vi "VI Linearisierung v2.vi"() -> ()   [LabVIEW 2020, in "Linearisierung v2.lvlib"] (continued)
                      n1878 = call "Komponentenindex aus SPAN.vi"("Component Index in"=w3418, "SPAN Idx in (Eingang)"=w3419, "SpanInletClusterArray in (Eingang)"=w3420) -> ("Component Index out"=w3403:i32, "SPAN Idx out"=w3404:i32, "Komponenten Index"=w3417:u16)  [unwired: 5 in, 1 out]
                      n1879 = Bundle("SPAN Idx out"=w3404, "Component Index out"=w3403) -> (w3402:T219)  [unwired: 1 in]
                      n1880 = Equal?(x=w3413, y=w3412) -> (x = y?=w3406:bool)
                      n1881 = Bundle(w3413, w3402) -> (w3405:T220)  [unwired: 1 in]
                      n1882 = Bundle(w3406, w3406, "Gesamtkonzentration"=w3408, "höchste Konzentration Teilkomponente"=w3407) -> (w3409:T221)  [unwired: 1 in]
                      n1883 = call "Stufen abfragen Tabelle setzen und auslesen.vi"("E/A Cluster"=w3409, "Ausgabetabelle (Eingang)"=w3410, "GD Cluster"=w3414, "Eingabetabelle (Eingang)"=w3411, "Fehler (Eingang, kein Fehler)"=w3421, "Komponente in"=w3417, "Index Cluster"=w3405, "GD in"=w3416) -> ("Fehler (Ausgang)"=w3415:errorcluster, "EGAK out"=w3422:T26[], "Stufen Tabellen out"=w3423:string[][])  [unwired: 1 out]
                    }
                  }
                }
                n1884 = Decrement(x=w3324) -> ()  [unwired: 1 out]
                n1885 = call "Komponentenindex aus SPAN.vi"("Component Index in"=w3301, "SPAN Idx in (Eingang)"=w3321, "SpanInletClusterArray in (Eingang)"=w3322) -> ("Summenformel"=w3305:T12)  [unwired: 5 in, 3 out]
                n1886 = call "set Tables Flag from SPANIdx.vi"("SPAN Idx"=w3302) -> ("set Tables"=w3304:bool)  [unwired: 10 in]
                n1887 = property class="Tbl (strikt)"(reference=w3357, "Value"=w3360) -> (error out=w3362:errorcluster)  [unwired: 1 in, 1 out]
                n1888 = property class="Arr (strikt)"(reference=w3367, error in=w3334, "Value"=w3359) -> (error out=w3361:errorcluster)  [unwired: 1 out]
                n1889 = property class="Str (strikt)"(reference=w3325, "Value"=w3305) -> (error out=w3315:errorcluster)  [unwired: 1 in, 1 out]
                n1890 = flat-sequence {
                  tunnel: w3314 -> [_]
                  tunnel: w3313 -> [_]
                  tunnel: w3312 -> [_]
                  tunnel: w3304 -> [w3372]
                  tunnel: w3301 -> [w3371]
                  tunnel: w3303 -> [w3370]
                  tunnel: w3302 -> [w3369]
                  frame #0 {
                    # "#STB_keep"
                    n1891 = call "Set SPAN for Gasnumber Settings.vi"("set Tables"=w3372, "Component Index"=w3371, "SPNA index"=w3369, "Digital (Eingang)"=w3370) -> ()  [unwired: 7 in, 1 out]
                  }
                }
                n1892 = call <vilib>:"Clear Errors.vi"("error in (no error)"=w3362) -> ("error out"=w3314:errorcluster)  [unwired: 5 in, 1 out]
                n1893 = call <vilib>:"Clear Errors.vi"("error in (no error)"=w3361) -> ("error out"=w3313:errorcluster)  [unwired: 5 in, 1 out]
                n1894 = call <vilib>:"Clear Errors.vi"("error in (no error)"=w3315) -> ("error out"=w3312:errorcluster)  [unwired: 5 in, 1 out]
              }
              frame Error {
              }
            }
          }
        }
      }
      event "Punkte umkehren", "Punkte umkehren 2", "Punkte umkehren 3", "Punkte umkehren 4", "Punkte umkehren 5", "Punkte umkehren 6", "Punkte umkehren 7", "Punkte umkehren 8", "Punkte umkehren 9", "Punkte umkehren 10": Value Change {
        w3449 = T15 5 items=["LCD-Touch-Display", "Analog-Display", "AVL GDU", "Horiba GDC", "HovaCal", "Horiba 710 c"] ("x")
        # "#STB_keep"
        n1895 = event-data() -> ("CtlRef"=w3492:refnum<vi>)  [unwired: 1 in]
        n1896 = for {
          tunnel: w3489 -> [w3570] mode=indexing
          tunnel: [w3568] -> w3485 mode=indexing
          n1897 = property class="Bool. (strikt)"(reference=w3570) -> (error out=w3569:errorcluster, "Value"=w3568:bool)  [unwired: 1 in, 1 out]
          n1898 = call <vilib>:"Clear Errors.vi"("error in (no error)"=w3569) -> ()  [unwired: 5 in, 2 out]
        }
        n1899 = Search 1D Array(1D array=w3489, element=w3492) -> (index of element=w3435:i32)  [unwired: 1 in]
        n1900 = call "FGV SpanEinstellungen.vi"("Punkte umkehren"=w3485, "Aktion"=Aktion_FGV_SpanEinstellungen."Punkte umkehren") -> ("error out"=w3486:errorcluster)  [unwired: 5 in, 4 out]
        n1901 = call "FGV SpanEinstellungen.vi"("Aktion"=Aktion_FGV_SpanEinstellungen."speichern", "error in (no error)"=w3486) -> ("error out"=w3442:errorcluster)  [unwired: 5 in, 4 out]
        n1902 = call "FGV SpanEinstellungen.vi"("Aktion"=Aktion_FGV_SpanEinstellungen."lesen", "error in (no error)"=w3442) -> ("error out"=w3468:errorcluster, "SpanInletClusterArray out"=w3439:T19[])  [unwired: 5 in, 3 out]
        n1903 = call "get SPAN active components indices for GD.vi"("error in (no error)"=w3468, "SPAN Idx"=w3435, "SpanInletClusterArray in"=w3439) -> ("error out"=w3471:errorcluster, "aktive Komponenten GD Indices"=w3469:i32[], "SPAN Idx out"=w3470:i32, "SpanInletClusterArray out"=w3472:T19[], "aktive Komponenten Indices additional"=w3466:u16[])  [unwired: 1 in, 3 out]
        n1904 = Index Array(array=w3484, index=w3435) -> (element=w3483:refnum<vi>)
        n1905 = call "Get Gaskomponenten sorted by Concentration.vi"("Fehler (Eingang, kein Fehler)"=w3471, "Component Index"=w3469, "SPAN Idx in (Eingang)"=w3470, "SpanInletClusterArray in (Eingang)"=w3472) -> ("Component Index out"=w3467:i32[], "SPAN Idx out (Ausgang)"=w3464:i32, "SpanInletClusterArray out (Ausgang)"=w3465:T19[], "höchste Konzentration Teilkomponente"=w3445:dbl, "Gesamtkonzentration"=w3446:dbl)  [unwired: 2 in, 1 out]
        n1906 = property class="Tbl (strikt)"(reference=w3483) -> (reference out=w3491:refnum<vi>, error out=w3482:errorcluster, "Value"=w3477:T27)  [unwired: 1 in]
        n1907 = call "set Tables Flag from SPANIdx.vi"("SPAN Idx"=w3435) -> ("set Tables"=w3437:bool)  [unwired: 10 in]
        n1908 = Build Array (concatenate)(w3466, w3467) -> (w3463:i32[])
        n1909 = Array Size(array=w3463) -> (size(s)=w3478:i32)
        n1910 = Decrement(x=w3478) -> (x-1=w3454:i32)
        n1911 = call "Get Stufentabellen aller Gaskomponenten.vi"("Component Index"=w3463, "SPAN Idx in (Eingang)"=w3464, "SpanInletClusterArray in (Eingang)"=w3465) -> ("Component Index out"=w3475:i32[], "SPAN Idx out (Ausgang)"=w3473:i32, "SpanInletClusterArray out (Ausgang)"=w3474:T19[], "Stufen Tabelle Array"=w3479:string[][][])  [unwired: 3 in, 2 out]
        n1912 = Replace Array Subset(array=w3479, new element=w3477, index (dim 0)=w3454) -> (w3476:string[][][])  [unwired: 2 in]
        n1913 = for {
          tunnel: w3475 -> [w3548] mode=indexing
          tunnel: w3483 -> [w3552]
          tunnel: w3437 -> [w3551]
          tunnel: w3476 -> [w3549] mode=indexing
          shift-right: [w3542] -> w3457
          shift-left: w3482 -> [w3550]
          tunnel: [w3541] -> w3460
          tunnel: w3474 -> [w3547]
          tunnel: [w3544] -> w3462 mode=indexing
          tunnel: [w3543] -> w3459
          tunnel: [w3541] -> w3455 mode=indexing
          shift-right: [w3540] -> w3441
          shift-left: w3473 -> [w3546]
          tunnel: [w3539] -> w3440 mode=indexing
          n1914 = call "Komponentenindex aus SPAN.vi"("Component Index in"=w3548, "SPAN Idx in (Eingang)"=w3546, "SpanInletClusterArray in (Eingang)"=w3547) -> ("Component Index out"=w3539:i32, "SPAN Idx out"=w3540:i32, "Komponenten Index"=w3545:u16)  [unwired: 5 in, 1 out]
          n1915 = Index Array(array=w3549, index (col) #1=0 ("Deaktivierter Index (Spalte)"), index (col) #2=1 ("Index (Spalte)")) -> (element #1=w3560:string[], element #2=w3559:string[])  [unwired: 2 in]
          n1916 = case shown="True" w3551 {
            tunnel: w3545 -> [w3562 w3567]
            tunnel: w3552 -> [_ w3566]
            tunnel: [w3562 w3565] -> w3544
            tunnel: [w3561 w3564] -> w3542
            tunnel: w3550 -> [w3561 w3563]
            frame False {
            }
            frame True {
              n1917 = call "Stufen abfragen Tabelle vorbereiten.vi"("Fehler (Eingang)"=w3563, "Komponente in"=w3567, "Tabelle (Eingang)"=w3566) -> ("Fehler (Ausgang)"=w3564:errorcluster, "Komponente out"=w3565:u16)  [unwired: 6 in, 1 out]
            }
          }
          n1918 = Reverse 1D Array(array=w3560) -> (reversed array=w3558:string[])
          n1919 = Reverse 1D Array(array=w3559) -> (reversed array=w3557:string[])
          n1920 = Build Array(w3558, w3557) -> (w3556:string[][])
          n1921 = call "Lin Daten aufarbeiten.vi"("Index (Seite)"=w3544, "Aktionen"=Aktion_Lin_Daten_aufarbeiten."lesen") -> ("EKAG"=w3543:string[])  [unwired: 15 in, 10 out]
          n1922 = Transpose 2D Array(2D array=w3556) -> (transposed array=w3541:string[][])
        }
        n1923 = call "FGV Gasteiler.vi"("Aktionen"=Aktionen_FGV_Gasteiler_Daten."lesen") -> ("Gasteiler Daten"=w3450:T118)  [unwired: 11 in, 7 out]
        n1924 = Unbundle By Name(w3450) -> ("Gasteiler Type"=w3451:T15)
        n1925 = Bundle(cluster=T157 {"Stufen Tabellen in"=[], "EGAK"=[], "AGAK"=[]} ("GD in"), "Stufen Tabellen in"=w3455, "EGAK"=w3459) -> (w3458:T157)  [unwired: 1 in]
        n1926 = Equal?(x=w3449, y=w3451) -> (x = y?=w3448:bool)
        n1927 = Bundle(w3448, FALSE) -> (w3444:cluster{bool, bool})  [unwired: 1 in]
        n1928 = case shown="True" w3437 {
          tunnel: w3458 -> [w3500 w3517]
          tunnel: w3462 -> [w3497 w3520]
          tunnel: w3457 -> [w3499 w3519]
          tunnel: [w3498 w3518] -> w3461
          tunnel: w3454 -> [_ w3516]
          tunnel: w3453 -> [_ w3515]
          tunnel: w3452 -> [_ w3514]
          tunnel: w3444 -> [_ w3513]
          tunnel: w3446 -> [_ w3512]
          tunnel: w3445 -> [_ w3511]
          tunnel: w3441 -> [w3496 w3510]
          tunnel: w3440 -> [w3495 w3509]
          frame False {
            n1929 = for {
              tunnel: w3500 -> [w3508]
              tunnel: w3497 -> [w3505] mode=indexing
              shift-right: [w3506] -> w3498
              shift-left: w3499 -> [w3507]
              tunnel: w3496 -> [w3503]
              tunnel: w3495 -> [w3502] mode=indexing
              i -> [w3504]
              n1930 = Bundle("SPAN Idx out (Ausgang)"=w3503, "Component Index out"=w3502) -> (w3501:T222)  [unwired: 1 in]
              n1931 = call "set Stufentabelle.vi"("Index in"=w3501, "Fehler (Eingang, kein Fehler)"=w3507, "Komponente in"=w3505, "Table Index"=w3504, "GD in"=w3508) -> ("Fehler (Ausgang)"=w3506:errorcluster)  [unwired: 3 in, 3 out]
            }
          }
          frame True {
            n1932 = for {
              tunnel: w3520 -> [w3538] mode=indexing
              tunnel: w3517 -> [w3535]
              shift-right: [w3536] -> w3518
              shift-left: w3519 -> [w3537]
              tunnel: w3516 -> [w3533]
              tunnel: w3515 -> [w3532]
              tunnel: w3514 -> [w3531]
              tunnel: w3513 -> [w3530]
              tunnel: w3512 -> [w3528]
              tunnel: w3511 -> [w3527]
              tunnel: w3510 -> [w3523]
              tunnel: w3509 -> [w3521] mode=indexing
              i -> [w3534]
              n1933 = Bundle("SPAN Idx out (Ausgang)"=w3523, "Component Index out"=w3521) -> (w3522:T222)  [unwired: 1 in]
              n1934 = Equal?(x=w3534, y=w3533) -> (x = y?=w3526:bool)
              n1935 = Bundle(w3534, w3522) -> (w3524:T223)  [unwired: 1 in]
              n1936 = Bundle(w3526, FALSE, "Gesamtkonzentration"=w3528, "höchste Konzentration Teilkomponente"=w3527) -> (w3529:T221)  [unwired: 1 in]
              n1937 = call "Stufen abfragen Tabelle setzen und auslesen.vi"("E/A Cluster"=w3529, "Ausgabetabelle (Eingang)"=w3531, "GD Cluster"=w3530, "Eingabetabelle (Eingang)"=w3532, "Fehler (Eingang, kein Fehler)"=w3537, "Komponente in"=w3538, "Index Cluster"=w3524, "GD in"=w3535) -> ("Fehler (Ausgang)"=w3536:errorcluster)  [unwired: 3 out]
            }
          }
        }
        n1938 = property class="Tbl (strikt)"(reference=w3491, error in=w3461, "Value"=w3460) -> (error out=w3490:errorcluster)  [unwired: 1 out]
        n1939 = call <vilib>:"Clear Errors.vi"("error in (no error)"=w3490) -> ("error out"=w3438:errorcluster)  [unwired: 5 in, 1 out]
        n1940 = call "Set SPAN for Gasnumber Settings.vi"("set Tables"=w3437, "error in (no error)"=w3438, "Component Index"=0 ("Component Index in"), "SPNA index"=w3435, "Digital (Eingang)"=w3436) -> ()  [unwired: 6 in, 1 out]
      }
      event Value Change {
        w3577 = FALSE  # automatisch
        n1941 = event-data() -> ()  [unwired: 1 in, 1 out]
        n1942 = call "Komponentenausgabe.vi"() -> ("error out"=w3572:errorcluster, "Gaskomponente"=w3573:T7)  [unwired: 8 in, 2 out]
        n1943 = call "Alle Rohdaten abholen.vi"("automatisch"=w3577, "error in (no error)"=w3572, "Temp. Messzelle G-nr."=w3574, "Gasindex"=w3573) -> ("error out"=w3576:errorcluster, "Gasindex out"=w3571:i32)  [unwired: 6 in]
        n1944 = call "Lin Daten aufarbeiten.vi"("Index (Seite)"=w3571, "error in (no error)"=w3576, "Aktionen"=Aktion_Lin_Daten_aufarbeiten."lesen") -> ("Eingabetabelle"=w3581:T54, "error out"=w3575:errorcluster)  [unwired: 14 in, 9 out]
        n1945 = call "AusgabeTabelle zusammenbauen.vi"("error in (no error)"=w3575, "Eingabetabelle"=w3581) -> ("Eingabetabelle behandelt"=w3580:string[][], "Ausgabetabelle"=w3583:T53)  [unwired: 7 in, 1 out]
        n1946 = local write "Ausgabetabelle"(w3583) -> ()
        n1947 = local write "Eingabetabelle"(w3580) -> ()
      }
      event Shortcut Menu Selection (User) {
        n1948 = event-data() -> ("ItemTag"=w3603:string)  [unwired: 1 in]
        n1949 = call "Editierte Zelle merken.vi"("Aktion"=enum16{"init", "lesen", "schreiben"}."lesen") -> ("Row"=w3601:i32)  [unwired: 9 in, 1 out]
        n1950 = case shown="\"Zeile davor einfügen\"" w3603 {
          tunnel: w3601 -> [_ w3604 w3607]
          tunnel: [_ w3605 w3608] -> w3597
          frame "False", Default {
          }
          frame "Zeile löschen" {
            n1951 = call "Lin Daten aufarbeiten.vi"("Zeile"=w3604, "Aktionen"=Aktion_Lin_Daten_aufarbeiten."Zeile löschen") -> ("error out"=w3605:errorcluster)  [unwired: 15 in, 10 out]
          }
          frame "Zeile davor einfügen" {
            n1952 = call "Lin Daten aufarbeiten.vi"("Zeile"=w3607, "Aktionen"=Aktion_Lin_Daten_aufarbeiten."Zeile einfügen") -> ("error out"=w3608:errorcluster)  [unwired: 15 in, 10 out]
          }
        }
        n1953 = call "Komponentenausgabe.vi"() -> ("Gaskomponente"=w3587:T7)  [unwired: 8 in, 3 out]
        n1954 = call "Lin Daten aufarbeiten.vi"("Index (Seite)"=w3587, "error in (no error)"=w3597, "Aktionen"=Aktion_Lin_Daten_aufarbeiten."EPA auswerten") -> ("Index (Seite) out"=w3588:i32, "error out"=w3598:errorcluster)  [unwired: 14 in, 9 out]
        n1955 = call "Lin Daten aufarbeiten.vi"("Index (Seite)"=w3588, "error in (no error)"=w3598, "Polynom-Ordnung"=Auswahl_Polynom_Ordnung."actual", "Aktionen"=Aktion_Lin_Daten_aufarbeiten."Lin auswerten") -> ("Index (Seite) out"=w3586:i32, "error out"=w3591:errorcluster)  [unwired: 13 in, 9 out]
        n1956 = call "Lin Daten aufarbeiten.vi"("Index (Seite)"=w3586, "error in (no error)"=w3591, "Aktionen"=Aktion_Lin_Daten_aufarbeiten."lesen") -> ("Eingabetabelle"=w3595:T54, "error out"=w3596:errorcluster)  [unwired: 14 in, 9 out]
        n1957 = call "AusgabeTabelle zusammenbauen.vi"("error in (no error)"=w3596, "Eingabetabelle"=w3595) -> ("Eingabetabelle behandelt"=w3592:string[][], "Ausgabetabelle"=w3593:T53)  [unwired: 7 in, 1 out]
        n1958 = local write "Ausgabetabelle"(w3593) -> ()
        n1959 = local write "Eingabetabelle"(w3592) -> ()
      }
      event Value Change {
        w3631 = u16 0 items=["---", "NO (350,3000) LP 191C", "NO2 (150) LP 191C (1of2)", "NO2 (2000) LP 191C (2of2)", "N2O (300) LP 191C (1of2)", "NH3 (300) LP 191C (1of2)", "NH3 (900,3000) LP 191C (2of2)", "HNCO (400) 191C", "H2O% (30) LP 191C", "Formaldehyde (70,500) LP 191C", "CO2 low% (4) LP 191C (2of2)", "CO2% (20) LP 191C (1of2)", "CO (700) LP 191C (1of3)", "CO% (1) LP 191C (2of3)", "Propylene (1000) LP 191C", "Aromatic HC C7 (500) LP 191C", "Ethylene (1000) LP 191C", "CH4 (250) LP 191C (1of2)", "CH4 (5000) LP 191C (2of2)", "Ethane (1000) LP 191C", "Acetylene (1000) LP 191C", "HNO2 (20) 191C", "MeOH (1000) 191C", "CO% (10) LP 191C (3of3)", "Formic Acid (100) 191C", "SO2 (500) LP 191C", "Acetaldehyde (1000) LP 191C", "COS (100) LP 191C", "1,3 butadiene (100) LP 191C", "Oil as Octane (200) LP 191C", "N2O (1000) LP 191C (2of2)", "Propane (200) LP 191C", "NO2 autorange (2000)", "CO autorange (100000)", "CH4 autorange (5000)", "NH3 autorange (3000)", "NOx autorange (3000)", "HCD (10000)", "NMHCD (10000)", "CO2% autorange (20)", "H2Oppm (300000)", "N2O autorange (1000)", "NMNEHCD (3000)", "Temp. Gascell", "Pressure Gascell", "sBeam@2500", "Temp. HL zu FT-IR", "Temp. HL Extern SP1", "Austrittstemp. FT-IR", "Temp. Schaltschrank", "Konstant 0", "Konstant 50", "Konstant 100", "AK DUMMY"] ("passive Komponente:")
        # "#LIN_only_saved_Polynoms"
        # "#PDF_manu_MG"
        # "#Option10xSpanAuto #LinEinheiten"
        n1960 = event-data() -> ("CtlRef"=w3624:refnum<vi>, "OldVal"=w3623:T49, "NewVal"=w3622:T49)  [unwired: 1 in]
        n1961 = call "FGV Spans abarbeiten.vi"("Aktion"=Aktion_FGV_Spans_abarbeiten."lesen") -> ("active SPAN Idx out"=w3639:i32)  [unwired: 5 in, 5 out]
        n1962 = call "FGV SpanEinstellungen.vi"("Aktion"=Aktion_FGV_SpanEinstellungen."lesen") -> ("automatisch out"=w3633:T20)  [unwired: 6 in, 4 out]
        n1963 = control-ref of="Gasnummer Generieren"() -> (w3629:refnum<vi>)
        n1964 = call "FGV Gasteiler.vi"("Aktionen"=Aktionen_FGV_Gasteiler_Daten."lesen") -> ("Aufzeichnung Start"=w3640:bool)  [unwired: 11 in, 7 out]
        n1965 = Less Than 0?(x=w3639) -> (x < 0?=w3638:bool)
        n1966 = Not(x=w3633) -> (.not. x?=w3632:T20)
        n1967 = Equal?(x=w3629, y=w3624) -> (x = y?=w3628:bool)
        n1968 = call "Komponentenausgabe HovaCAL fix.vi"("Gasnummer in"=w3622) -> ("fix"=w3626:bool, "Gaskomponente"=w3625:T7, "Gasnummer out"=w3627:T49)  [unwired: 7 in, 1 out]
        n1969 = Or(x=w3638, y=w3632) -> (x .or. y?=w3634:T20)
        n1970 = Not(x=w3640) -> (.not. x?=w3636:bool)
        n1971 = And(x=w3634, y=w3636) -> (x .and. y?=w3637:T20)
        n1972 = And(x=w3628, y=w3626) -> (x .and. y?=w3630:bool)
        n1973 = case shown="False" w3630 {
          tunnel: w3627 -> [w3656 w3679]
          tunnel: [w3658 w3681] -> w3648
          tunnel: w3637 -> [w3657 _]
          tunnel: w3625 -> [_ w3681]
          tunnel: w3623 -> [_ w3680]
          tunnel: [w3656 w3680] -> w3619
          tunnel: [w3656 w3679] -> w3621
          tunnel: w3611 -> [w3655 _]
          tunnel: w3610 -> [w3654 _]
          frame False {
            n1974 = case shown="True" w3657 {
              tunnel: w3656 -> [w3660 w3663]
              tunnel: [w3661 w3668] -> w3658
              tunnel: w3655 -> [_ w3664]
              tunnel: w3654 -> [_ w3665]
              frame False {
                # "Gasnummer … in LIN Polynom immer … wegen Punkte abholen umschalten und anzeigen !\n(sollte sich in Protokoll nicht auswirken, weil GD schon läuft)"
                n1975 = call "Gasnummer in LIN Polynom setzen.vi"("Gasnummer"=w3660) -> ("Fehler (Ausgang)"=w3659:errorcluster)  [unwired: 8 in, 2 out]
                n1976 = call "Komponentenausgabe.vi"("error in (no error)"=w3659) -> ("Gaskomponente"=w3661:T7)  [unwired: 7 in, 3 out]
              }
              frame True {
                # "#LinV2_auto_singleSave"
                n1977 = control-ref of="Autolin Hovacal"() -> (w3671:refnum<vi>)
                n1978 = disable-structure shown="Aktiviert" {
                  disable-tunnel: [w3673 _] -> w3669
                  frame Disabled {
                    n1979 = call "FGV SpanEinstellungen.vi"("Aktion"=Aktion_FGV_SpanEinstellungen."lesen") -> ("automatisch out"=w3674:T20)  [unwired: 6 in, 4 out]
                    n1980 = Not(x=w3674) -> (.not. x?=w3673:T20)
                  }
                  frame Enabled {
                    # "MG ???"
                  }
                }
                n1981 = control-ref of="Daten"() -> (w3672:refnum<vi>)
                n1982 = call "Set SPAN Component.vi"("Protocol_only"=FALSE, "Gasnummer"=w3663, "Autolin Hovacal (alt)"=w3671, "Daten Hovacal (alt)"=w3672) -> ("Gaskomponente"=w3668:T7)  [unwired: 3 in, 4 out]
                n1983 = case shown="True" w3669 {
                  tunnel: w3668 -> [_ w3678]
                  frame False {
                  }
                  frame True {
                    n1984 = call "FGV Gasteilerliste laden.vi"("Aktion"=Aktion_FGV_Gasteilerliste_laden."Gas vereinzeln", "Gasindex"=w3678) -> ("Formel"=w3676:string)  [unwired: 7 in, 2 out]
                    n1985 = local write "PrüfgasName"(w3676) -> ()
                  }
                }
                n1986 = Decrement(x=w3663) -> (x-1=w3662:T49)
                n1987 = call "MG FileName.vi"("Gasnummer:"=w3662) -> ("LIN TXT Datei Name"=w3666:string, "EPA TXT Datei Name"=w3667:string)  [unwired: 7 in, 2 out]
                n1988 = call "Preset Filenames.vi"("FileNameInput References"=w3664, "Filename Flag Cluster"=w3665, "LIN TXT Datei Name"=w3666, "EPA TXT Datei Name"=w3667) -> ()  [unwired: 8 in]
              }
            }
          }
          frame True {
            # "#HovaCALMultiMFC \nHovaCAL Komponente fix\nnur für Daten aufzeichnen ..."
          }
        }
        n1989 = call "Einheiten finden.vi"("Komponente"=w3648) -> ("Einheit in String"=w3647:string)  [unwired: 6 in, 4 out]
        "Einheit" <- w3647
        "Einheit Deviation" <- w3647
        n1990 = local read "Hauptregisterkarte"() -> (w3653:T8)
        n1991 = local write "passive Komponente:"(w3631) -> ()
        n1992 = local write "Gasnummer HovaCal Interface"(w3619) -> ()
        n1993 = local write "Gasnummer HovaCal"(w3619) -> ()
        n1994 = local write "Gasnummer EPA"(w3619) -> ()
        n1995 = local write "Gasnummer LIN"(w3619) -> ()
        n1996 = local write "Gasnummer Generieren"(w3621) -> ()
        n1997 = Decrement(x=w3619) -> (x-1=w3613:T49)
        n1998 = call "aktueller SPAN und Komponent Index.vi"() -> ("akt SPAN out"=w3614:i32)  [unwired: 7 in, 4 out]
        n1999 = Bundle("akt SPAN out"=w3614, w3613) -> (w3612:cluster{"akt SPAN out":i32, T49})  [unwired: 1 in]
        n2000 = call "EPA Polynom Ordnung je Komponente für Protokoll.vi"("Aktion"=Aktion_EPA_Polynom_Ordnung_je_Komponente_für_Protokoll."lesen", "Index in"=w3612) -> ("EPA Optionsfeld out"=w3617:T2)  [unwired: 5 in, 3 out]
        n2001 = call "LIN Polynom Ordnung je Komponente für Protokoll.vi"("Aktion"=Aktion_LIN_Polynom_Ordnung_je_Komponente_für_Protokoll."lesen", "Index in"=w3612) -> ("Polynom-Ordnung view only out"=w3616:T55)  [unwired: 3 in, 6 out]
        n2002 = case shown="\"Span Einstellungen\", Standard" w3653 {
          tunnel: w3648 -> [w3689 w3694 w3713 w3743]
          tunnel: [w3690 w3706 w3727 w3754] -> w3652
          tunnel: [w3688 w3704 w3726 w3753] -> w3651
          tunnel: w3647 -> [w3684 w3703 w3722 w3747]
          tunnel: w3646 -> [w3682 w3700 _ _]
          tunnel: w3645 -> [_ _ _ w3746]
          tunnel: w3644 -> [_ _ w3721 _]
          tunnel: w3643 -> [w3683 w3701 _ _]
          tunnel: w3617 -> [_ _ w3715 _]
          tunnel: w3616 -> [_ _ _ w3738]
          frame "Span Einstellungen", Default {
            # "#MG_GK_back_calc"
            # "#Option10xSpanAuto\n\nGasnummer in Auto gesperrt, kann immer nur SPAN1 sein !"
            n2003 = call "Einheiten in Tabellenspalten.vi"("Einheit"=w3684, "Tabelle (Eingang)"=w3683) -> ("Einheit out"=w3685:string)  [unwired: 7 in, 2 out]
            n2004 = call "Einheiten in Tabellenspalten.vi"("Einheit"=w3685, "Tabelle (Eingang)"=w3682) -> ()  [unwired: 7 in, 3 out]
            n2005 = call "Lin Daten aufarbeiten.vi"("Index (Seite)"=w3689, "Aktionen"=Aktion_Lin_Daten_aufarbeiten."lesen") -> ("Aktiv EPA"=w3690:T57, "Aktiv LIN"=w3688:bool[], "Stufen Tabelle"=w3687:T27, "EKAG"=w3686:string[])  [unwired: 15 in, 7 out]
            n2006 = disable-structure shown="Deaktiviert" {
              disable-tunnel: w3687 -> [w3693 _]
              disable-tunnel: w3686 -> [w3692 _]
              frame Disabled {
                # "#STB_keep"
                n2007 = local write "Parameterkontrolle:"(w3692) -> ()
                n2008 = local write "Stufen Tabelle"(w3693) -> ()
              }
              frame Enabled {
              }
            }
          }
          frame "Daten aufzeichnen" {
            # "#PDF_manu_MG"
            # "#LinEinheiten"
            n2009 = call "Einheiten in Tabellenspalten.vi"("Einheit"=w3703, "Tabelle (Eingang)"=w3701) -> ("error out"=w3699:errorcluster, "Einheit out"=w3702:string)  [unwired: 7 in, 1 out]
            n2010 = call "Einheiten in Tabellenspalten.vi"("error in (no error)"=w3699, "Einheit"=w3702, "Tabelle (Eingang)"=w3700) -> ()  [unwired: 6 in, 3 out]
            n2011 = call "Lin Daten aufarbeiten.vi"("Index (Seite)"=w3694, "Aktionen"=Aktion_Lin_Daten_aufarbeiten."lesen") -> ("Aktiv EPA"=w3706:T57, "Aktiv LIN"=w3704:bool[], "Eingabetabelle"=w3708:T54, "Lin-Polynom"=w3695:T119)  [unwired: 15 in, 7 out]
            n2012 = call "Component Get Daten aufzeichnen.vi"("Lin-Polynom"=w3695, "Gaskomponente"=w3694) -> ("Autorange Offsets"=→"Offset":string, "Autorange Spanfactors"=→"Spanfactor":string, "Polynome"=w3698:T184)  [unwired: 6 in, 1 out]
            n2013 = call "AusgabeTabelle zusammenbauen.vi"("Eingabetabelle"=w3708) -> ("Eingabetabelle behandelt"=w3705:string[][], "Ausgabetabelle"=w3707:T53)  [unwired: 8 in, 1 out]
            n2014 = local write "Eingabetabelle"(w3705) -> ()
            n2015 = local write "Ausgabetabelle"(w3707) -> ()
            n2016 = local write "Polynom"(w3698) -> ()
          }
          frame "EPA 1065-307" {
            # "#PDF_manu_MG"
            # "#LinEinheiten"
            n2017 = call "Einheiten in Tabellenspalten.vi"("Einheit"=w3722, "Tabelle (Eingang)"=w3721) -> ()  [unwired: 7 in, 3 out]
            n2018 = call "Lin Daten aufarbeiten.vi"("Index (Seite)"=w3713, "Aktionen"=Aktion_Lin_Daten_aufarbeiten."lesen") -> ("Index (Seite) out"=w3712:i32, "Lin-Polynom"=w3710:T119, "error out"=w3711:errorcluster)  [unwired: 15 in, 8 out]
            n2019 = Bundle By Name(cluster=w3710, "EPA Optionsfeld"=w3715) -> (w3718:T119)
            n2020 = call "Lin Daten aufarbeiten.vi"("Index (Seite)"=w3712, "Lin-Polynom"=w3718, "error in (no error)"=w3711, "Aktionen"=Aktion_Lin_Daten_aufarbeiten."Protkolldaten") -> ("Index (Seite) out"=w3716:i32, "error out"=w3717:errorcluster)  [unwired: 13 in, 9 out]
            n2021 = call "Lin Daten aufarbeiten.vi"("Index (Seite)"=w3716, "error in (no error)"=w3717, "Aktionen"=Aktion_Lin_Daten_aufarbeiten."EPA auswerten") -> ("Index (Seite) out"=w3720:i32, "error out"=w3735:errorcluster)  [unwired: 14 in, 9 out]
            n2022 = call "Lin Daten aufarbeiten.vi"("Index (Seite)"=w3720, "error in (no error)"=w3735, "Aktionen"=Aktion_Lin_Daten_aufarbeiten."lesen") -> ("Aktiv EPA"=w3727:T57, "Aktiv LIN"=w3726:bool[], "Eingabetabelle"=w3733:T54, "EPA Auswertung"=w3723:cluster{sgl[], sgl[], bool[]}, "error out"=w3734:errorcluster)  [unwired: 14 in, 6 out]
            n2023 = call "EPA_Tabelle zusammenbauen.vi"("error in (no error)"=w3734, "Eingabetabelle"=w3733) -> ("error out"=w3732:errorcluster, "XY-Graph"=w3729:cluster{dbl[], dbl[]}[], "EPA Ausgabetabelle"=w3730:string[][])  [unwired: 7 in]
            n2024 = call "FGV Auswertung sammeln.vi"("Aktion"=Aktion_FGV_Auswertung_sammeln."lesen", "error in (no error)"=w3732) -> ("LINVer Auswertung"=w3728:string[][])  [unwired: 7 in, 2 out]
            n2025 = control-ref of="EPA Auswertung"() -> (w3725:refnum<vi>)
            n2026 = local write "EPA Auswertung"(w3728) -> ()
            n2027 = local write "EPA Ausgabetabelle"(w3730) -> ()
            n2028 = local write "XY-Graph EPA"(w3729) -> ()
            n2029 = Unbundle(w3723) -> (w3724:bool[])  [unwired: 2 out]
            n2030 = call "Zellen einfaerben.vi"("Färben"=w3724, "Tabellenref."=w3725) -> ()  [unwired: 10 in]
          }
          frame "LIN Anpassung" {
            # "#PDF_manu_MG"
            # "#LinEinheiten #AutorangeSpanfactorsOffsets"
            n2031 = call "Einheiten in Tabellenspalten.vi"("Einheit"=w3747, "Tabelle (Eingang)"=w3746) -> ()  [unwired: 7 in, 3 out]
            n2032 = call "Get Autorange Bereiche.vi"("Gaskomponente"=w3743) -> ("Autorange Bereiche"=w3744:T7[])  [unwired: 8 in, 2 out]
            n2033 = call "Lin Daten aufarbeiten.vi"("Index (Seite)"=w3743, "Polynom-Ordnung"=w3738, "Aktionen"=Aktion_Lin_Daten_aufarbeiten."Lin auswerten") -> ("Index (Seite) out"=w3745:i32, "error out"=w3751:errorcluster)  [unwired: 14 in, 9 out]
            n2034 = call "Lin Daten aufarbeiten.vi"("Index (Seite)"=w3745, "error in (no error)"=w3751, "Aktionen"=Aktion_Lin_Daten_aufarbeiten."lesen") -> ("Aktiv EPA"=w3754:T57, "Aktiv LIN"=w3753:bool[], "Eingabetabelle"=w3758:T54, "Lin-Polynom"=w3748:T119, "error out"=w3756:errorcluster)  [unwired: 14 in, 6 out]
            n2035 = Unbundle By Name(w3748) -> ("Polynomkoeff."=w3749:dbl[], "Spanfactors"=w3740:sgl[], "Offsets"=w3739:sgl[])
            n2036 = call "LinTabelle zusammenbauen.vi"("error in (no error)"=w3756, "Eingabetabelle"=w3758) -> ("LIN Ausgabetabelle"=w3755:string[][])  [unwired: 6 in, 3 out]
            n2037 = Array To Cluster(array=w3749) -> (cluster=w3750:T185)
            n2038 = call "Get Autorange Spanfactors and Offsets.vi"("Autorange Bereiche"=w3744, "Offset"=w3739, "Span"=w3740) -> ("Autorange Offsets"=→"Offset LIN":string, "Autorange Spanfactors"=→"Spanfactor LIN":string)  [unwired: 4 in, 3 out]
            n2039 = local write "LIN Ausgabetabelle"(w3755) -> ()
            n2040 = local write "LIN Polynomkoeffizienten"(w3750) -> ()
          }
        }
        n2041 = local write "EPA Optionsfeld"(w3617) -> ()
        n2042 = local write "Polynom-Ordnung"(w3616) -> ()
        n2043 = local write "Aktiv"(w3652) -> ()
        n2044 = local write "Aktiv LIN"(w3651) -> ()
      }
      event "HovaCAL MFC1 Komponente:", "HovaCAL MFC2 Komponente:", "HovaCAL MFC3 Komponente:", "HovaCAL MFC4 Komponente:", "HovaCAL MFC5 Komponente:", "HovaCAL Pump1 Komponente:", "HovaCAL Pump2 Komponente:": Value Change {
        # "#ReducePumpMFC"
        # "Konzentration übernehmen aber Sollwert schreiben erst beim Start  ..."
        # "Komponentenauswahl ergänzen !\npassiert nur bei der Auswahl ..."
        n2045 = event-data() -> ("CtlRef"=w3772:refnum<vi>)  [unwired: 1 in]
        n2046 = call "FGV_HovaCAL_Interface_ControlReferenzen.vi"("Aktion"=enum16{"lesen", "schreiben"}."lesen") -> ("MFC fix Cluster out"=w3773:T224)  [unwired: 6 in, 4 out]
        n2047 = Unbundle By Name(w3773) -> ("MFC Komponenten Array"=w3770:refnum<vi>[])
        n2048 = property class="Ring (strikt)"(reference=w3772) -> ("Strings []"=w3771:string[], "Value"=w3762:u16)  [unwired: 1 in, 2 out]
        n2049 = Search 1D Array(1D array=w3770, element=w3772) -> (index of element=w3769:i32)  [unwired: 1 in]
        n2050 = Build Array("HovaCAL MFC1 Komponente:", "HovaCAL MFC2 Komponente:", "HovaCAL MFC3 Komponente:", "HovaCAL MFC4 Komponente:", "HovaCAL MFC5 Komponente:", "HovaCAL Pump1 Komponente:", "HovaCAL Pump2 Komponente:") -> (w3775:u16[])
        n2051 = call "Reduce maxMFC 2 MFC count index for Pump index.vi"("MFC idx"=w3769) -> ("Pump"=w3763:bool, "Pump Idx"=w3764:i32, "AutoLin MFC"=w3767:i32)  [unwired: 8 in]
        n2052 = call "FGV_HovaCAL_Interface_AutoLin_MFC.vi"("Aktion"=Aktion_FGV_HovaCAL_Interface_Autolin."MFC Komponente fix setzen", "MFV Komponente fix"=w3775) -> ("error out"=w3766:errorcluster)  [unwired: 6 in, 3 out]
        n2053 = Equal To 0?(x=w3762) -> (x = 0?=w3761:bool)
        n2054 = case shown="False" w3761 {
          selector: w3761 -> [w3786 w3796]
          tunnel: w3771 -> [w3795 _]
          tunnel: w3762 -> [w3792 _]
          tunnel: [w3788 0.0 ("f")] -> w3768
          tunnel: [w3787 _] -> w3765
          tunnel: [w3786 w3796] -> w3760
          frame False {
            n2055 = Decrement(x=w3792) -> (x-1=w3791:u16)
            n2056 = Index Array(array=w3795, index=w3792) -> (element=w3787:string)
            n2057 = call "Komponent Konzentration mit Name finden.vi"("Komponente"=w3787) -> ("found"=w3794:bool, "Konzentration OUT"=w3790:dbl)  [unwired: 8 in, 1 out]
            n2058 = call "HovaCAL ppm convert from Component.vi"("Konzentration"=w3790, "Gasnummer"=w3791) -> ("Konzentration in ppm"=w3789:dbl)  [unwired: 5 in, 4 out]
            n2059 = Select(t=w3789, s=w3794, f=0.0) -> (s? t:f=w3788:dbl)
          }
          frame True {
          }
        }
        n2060 = case shown="True" w3763 {
          tunnel: w3766 -> [w3803 _]
          tunnel: w3768 -> [w3799 _]
          tunnel: w3767 -> [w3800 w3804]
          tunnel: w3765 -> [_ w3811]
          tunnel: w3764 -> [_ w3810]
          tunnel: w3760 -> [_ _]
          frame False {
            n2061 = call "HovaCAL_Interface_SetComponentConcentration.vi"("error in (no error)"=w3803, "AutoLin MFV Index"=w3800, "Konzentration"=w3799) -> ("error out"=w3802:errorcluster, "AutoLin MFV Index out"=w3801:u32, "Konzentration out"=w3798:dbl)  [unwired: 6 in]
            n2062 = call "HovaCAL_Interface_SetPoint.vi"("error in (no error)"=w3802, "AutoLin MFC Index"=w3801, "Konzentration"=w3798) -> ()  [unwired: 8 in, 1 out]
          }
          frame True {
            # "water/reagent"
            n2063 = call "HovaCAL_Interface_SetPumpParameter.vi"("Pump Idx"=w3810, "Komponent Name"=w3811) -> ("error out"=w3806:errorcluster)  [unwired: 9 in]
            n2064 = call "HovaCAL_Interface_SetComponentConcentration.vi"("error in (no error)"=w3806, "AutoLin MFV Index"=w3804, "Konzentration"=0.0) -> ("error out"=w3809:errorcluster, "AutoLin MFV Index out"=w3808:u32)  [unwired: 6 in, 1 out]
            n2065 = call "HovaCAL_Interface_SetPoint.vi"("error in (no error)"=w3809, "AutoLin MFC Index"=w3808, "Konzentration"=0.0) -> ()  [unwired: 8 in, 1 out]
          }
        }
      }
      event "fix+MFC1", "fix+MFC2", "fix+MFC3", "fix+MFC4", "fix+MFC5", "fix+Pump1", "fix+Pump2": Value Change {
        # "#ReducePumpMFC"
        n2066 = event-data() -> ("CtlRef"=w3833:refnum<vi>)  [unwired: 1 in, 5 out]
        n2067 = call "FGV_HovaCAL_Interface_ControlReferenzen.vi"("Aktion"=enum16{"lesen", "schreiben"}."lesen") -> ("MFC fix Cluster out"=w3827:T224)  [unwired: 6 in, 4 out]
        n2068 = Unbundle By Name(w3827) -> ("MFC Komponenten Array"=w3825:refnum<vi>[], "MFC fix + Array"=w3826:refnum<vi>[])
        n2069 = Search 1D Array(1D array=w3826, element=w3833) -> (index of element=w3824:i32)  [unwired: 1 in]
        n2070 = Index Array(array=w3825, index=w3824) -> (element=w3832:refnum<vi>)
        n2071 = call "FGV_HovaCAL_Interface_SetData.vi"("Aktion"=Aktion_FGV_HovaCAL_Interface_SetData."lesen") -> ("Set Values Cluster out"=w3830:T168)  [unwired: 8 in, 6 out]
        n2072 = property class="Ring (strikt)"(reference=w3832) -> ("Strings []"=w3837:string[], "Value"=w3822:u16)  [unwired: 1 in, 2 out]
        n2073 = Index Array(array=w3830, index=w3824) -> (element=w3829:T170)
        n2074 = Unbundle By Name(w3829) -> ("input concentration setpoint"=w3820:dbl)
        n2075 = Index Array(array=w3837, index=w3822) -> (element=w3814:string)
        n2076 = call "FGV_HovaCAL_Interface_AutoLin_MFC.vi"("Aktion"=Aktion_FGV_HovaCAL_Interface_Autolin."lesen") -> ("error out"=w3838:errorcluster)  [unwired: 7 in, 3 out]
        n2077 = Decrement(x=w3822) -> (x-1=w3821:u16)
        n2078 = call "HovaCAL ppm convert from Component.vi"("Konzentration"=w3820, "Gasnummer"=w3821) -> ("Konzentration in %"=w3819:dbl, "Gasnummer out"=w3818:T7)  [unwired: 5 in, 3 out]
        n2079 = call "Komponent Konzentration mit Name finden.vi"("Konzentration IST in"=w3819, "Komponente"=w3814) -> ("found"=w3835:bool, "Konzentration OUT"=w3817:dbl)  [unwired: 7 in, 1 out]
        n2080 = call "Reduce maxMFC 2 MFC count index for Pump index.vi"("MFC idx"=w3824) -> ("Pump"=w3815:bool, "Pump Idx"=w3813:i32, "AutoLin MFC"=w3823:i32)  [unwired: 8 in]
        n2081 = call "HovaCAL ppm convert from Component.vi"("Konzentration"=w3817, "Gasnummer"=w3818) -> ("Konzentration in ppm"=w3816:dbl)  [unwired: 5 in, 4 out]
        n2082 = Select(t=w3816, s=w3835, f=0.0) -> (s? t:f=w3836:dbl)
        n2083 = case shown="False" w3815 {
          tunnel: w3838 -> [w3847 _]
          tunnel: w3836 -> [w3843 _]
          tunnel: w3823 -> [w3842 _]
          tunnel: w3814 -> [_ _]
          tunnel: w3813 -> [_ _]
          frame False {
            n2084 = call "HovaCAL_Interface_SetComponentConcentration.vi"("error in (no error)"=w3847, "AutoLin MFV Index"=w3842, "Konzentration"=w3843) -> ("error out"=w3846:errorcluster, "AutoLin MFV Index out"=w3845:u32)  [unwired: 6 in, 1 out]
            n2085 = call "HovaCAL_Interface_SetPoint.vi"("error in (no error)"=w3846, "AutoLin MFC Index"=w3845, "Konzentration"=0.0) -> ()  [unwired: 8 in, 1 out]
          }
          frame True {
            # "water/reagent"
          }
        }
      }
      event "passive Komponente:": Value Change {
        n2086 = event-data() -> ()  [unwired: 1 in, 1 out]
        n2087 = call "Komponentenausgabe.vi"() -> ("Gaskomponente"=w3856:T7)  [unwired: 8 in, 3 out]
        n2088 = Decrement(x="passive Komponente:") -> (x-1=w3857:u16)
        n2089 = Equal To 0?(x="passive Komponente:") -> (x = 0?=w3859:bool)
        n2090 = Select(t=w3856, s=w3859, f=w3857) -> (s? t:f=w3853:T7)
        n2091 = call "Einheiten finden.vi"("Komponente"=w3853) -> ("Einheit in String"=w3851:string)  [unwired: 6 in, 4 out]
        n2092 = call "Lin Daten aufarbeiten.vi"("Index (Seite)"=w3853, "Aktionen"=Aktion_Lin_Daten_aufarbeiten."lesen") -> ("Eingabetabelle"=w3861:T54)  [unwired: 15 in, 10 out]
        n2093 = call "AusgabeTabelle zusammenbauen.vi"("Eingabetabelle"=w3861) -> ("Eingabetabelle behandelt"=w3854:string[][], "Ausgabetabelle"=w3855:T53)  [unwired: 8 in, 1 out]
        n2094 = call "Einheiten in Tabellenspalten.vi"("Einheit"=w3851, "Tabelle (Eingang)"=w3850) -> ("Einheit out"=w3852:string)  [unwired: 7 in, 2 out]
        n2095 = local write "Ausgabetabelle"(w3855) -> ()
        n2096 = local write "Eingabetabelle"(w3854) -> ()
        n2097 = call "Einheiten in Tabellenspalten.vi"("Einheit"=w3852, "Tabelle (Eingang)"=w3849) -> ()  [unwired: 7 in, 3 out]
      }
      event Value Change {
        # "#Option10xSpanAuto"
        n2098 = event-data() -> ("NewVal"=w3866:T12, "CtlRef"=w3869:refnum<vi>)  [unwired: 1 in]
        n2099 = call "Komponentenausgabe.vi"() -> ("Gaskomponente"=w3867:T7)  [unwired: 8 in, 3 out]
        n2100 = Search 1D Array(1D array=w3870, element=w3869) -> (index of element=w3868:i32)  [unwired: 1 in]
        n2101 = call "FGV Gasteilerliste laden.vi"("Aktion"=Aktion_FGV_Gasteilerliste_laden."Formel ändern", "PrüfgasName"=w3866, "Gasindex"=w3867) -> ("error out"=w3875:errorcluster)  [unwired: 6 in, 2 out]
        n2102 = call "FGV Gasteilerliste laden.vi"("Aktion"=Aktion_FGV_Gasteilerliste_laden."Liste erstellen", "error in (no error)"=w3875) -> ("error out"=w3874:errorcluster)  [unwired: 7 in, 2 out]
        n2103 = call "FGV Gasteilerliste laden.vi"("Aktion"=Aktion_FGV_Gasteilerliste_laden."speichern", "error in (no error)"=w3874) -> ("error out"=w3865:errorcluster)  [unwired: 7 in, 2 out]
        n2104 = call "Set Summenformel.vi"("error in (no error)"=w3865, "Summenformel"=w3866, "Gaskomponente"=w3867, "SPAN Idx"=w3868) -> ()  [unwired: 7 in, 1 out]
      }
      event "HovaCAL AutoLin MFC": Value Change {
        w3906 = T15 4 items=["LCD-Touch-Display", "Analog-Display", "AVL GDU", "Horiba GDC", "HovaCal", "Horiba 710 c"] ("x")
        # "immer FALSE und damit erster (aktiver!) SPAN oder aktuell laufender im automatic Modus ??? ... im Automaitc Modus muss das gesperrt sein !!!\nAblaufdatum fehlt im Protokoll ?! -> ergänzt"
        # "#Option10xSpanAuto\n-> Gasnummer generieren"
        n2105 = event-data() -> ()  [unwired: 1 in, 1 out]
        n2106 = call "Lin Daten aufarbeiten.vi"("Aktionen"=Aktion_Lin_Daten_aufarbeiten."lesen") -> ("Lin-Polynom"=w3887:T119)  [unwired: 16 in, 10 out]
        n2107 = call "FGV SpanEinstellungen.vi"("Aktion"=Aktion_FGV_SpanEinstellungen."lesen") -> ("SpanInletClusterArray out"=w3920:T19[])  [unwired: 6 in, 4 out]
        n2108 = disable-structure shown="HovaCALInterface==TRUE, Standard" {
          disable-tunnel: ["HovaCAL AutoLin MFC" "Autolin Hovacal"] -> w3908
          frame condition #0 (active) {
          }
          frame condition #1 {
          }
        }
        n2109 = case shown="False" FALSE {
          tunnel: w3887 -> [w3971 w4001]
          tunnel: w3920 -> [w3972 _]
          tunnel: [w3984 w4000] -> w3919
          tunnel: [w3983 w3999] -> w3918
          tunnel: [w3982 w3998] -> w3917
          tunnel: [w3980 w3997] -> w3916
          tunnel: [w3979 w3996] -> w3915
          tunnel: [w3978 w3995] -> w3914
          tunnel: [w3977 w3994] -> w3913
          tunnel: [w3976 w3993] -> w3912
          tunnel: [w3975 w3992] -> w3911
          tunnel: [w3974 w3991] -> w3910
          tunnel: [w3973 w3990] -> w3909
          tunnel: [w3958 w3989] -> w3884
          tunnel: w3902 -> [w3961 _]
          tunnel: [w3959 w3988] -> w3901
          tunnel: [w3957 _] -> w3900
          tunnel: [w3956 w3987] -> w3894
          frame False {
            n2110 = Unbundle By Name(w3971) -> ("Gasnummer:"=w3954:u8)
            n2111 = call "get active SPAN.vi"("SpanInletClusterArray in"=w3972) -> ("Index active SPAN"=w3957:i32, "SpanInletClusterArray out"=w3970:T19[])  [unwired: 8 in, 1 out]
            n2112 = Index Array(array=w3961, index=w3957) -> (element=w3962:refnum<vi>)
            n2113 = call "get SPAN first active component.vi"("SPAN Idx"=w3957, "SpanInletClusterArray in"=w3970) -> ("first aktive Komponente"=w3963:i32, "SPAN Idx out"=w3966:i32, "SpanInletClusterArray out"=w3969:T19[])  [unwired: 6 in, 1 out]
            n2114 = property class="Bool. (strikt)"(reference=w3962) -> (error out=w3960:errorcluster, "Value"=w3959:bool)  [unwired: 1 in, 1 out]
            n2115 = Decrement(x=w3954) -> (x-1=w3951:u8)
            n2116 = Equal To 0?(x=w3954) -> (x = 0?=w3955:bool)
            n2117 = call "is SPAN component active.vi"("Komponente"=w3951, "SPAN Idx"=w3966, "SpanInletClusterArray in"=w3969) -> ("aktiv?"=w3965:bool, "SPAN Idx out"=w3967:i32, "SpanInletClusterArray out"=w3968:T19[])  [unwired: 5 in, 1 out]
            n2118 = Select(t=u8 1, s=w3955, f=w3954) -> (s? t:f=w3952:u8)
            n2119 = Increment(x=w3963) -> (x+1=w3964:i32)
            n2120 = call <vilib>:"Clear Errors.vi"("error in (no error)"=w3960) -> ()  [unwired: 5 in, 2 out]
            n2121 = Index Array(array=w3968, index=w3967) -> (element=w3986:T19)
            n2122 = Select(t=w3952, s=w3965, f=w3964) -> (s? t:f=w3958:i32)
            n2123 = Unbundle By Name(w3986) -> ("Konfig Gasflasche"=w3984:T20, "Gasflasche"=w3983:T22, "Komponenten"=w3985:T23, "Trägergas"=w3981:T26, "Gasflaschen Nr.:"=w3979:string, "Max Fehler"=w3977:sgl, "Zeitdauer Stufen"=w3976:sgl, "Anzahl Stufen"=w3975:sgl, "Analysator"=w3974:T21, "Ablaufdatum"=w3973:timestamp, "zusätzliche Zeitdauer Erster Punkt"=w3956:sgl)
            n2124 = call "Komponentenauswahl aus No1.vi"("Komponente 1"=w3985) -> ("Genauigkeit"=w3978:dbl, "Komponentenauswahl"=w3982:T217)  [unwired: 8 in, 1 out]
            n2125 = call "Verduennungsgas aus Traegergas.vi"("Trägergas"=w3981) -> ("Verdünnungsgas"=w3980:T121)  [unwired: 10 in]
          }
          frame True {
            n2126 = Unbundle By Name(w4001) -> ("Konfig Gasflasche"=w4000:T20, "Gasflasche"=w3999:T22, "Komponentenauswahl"=w3998:T120, "Verdünnungsgas"=w3997:T121, "Gasflaschen Nr.:"=w3996:string, "Bottle Accuracy"=w3995:dbl, "F_max gefordert (%)"=w3994:sgl, "Zeitdauer Stufe"=w3993:T122, "Anzahl Stufen"=w3992:T122, "Messgerät"=w3991:string, "Gas Ablaufdatum"=w3990:timestamp, "Gasnummer:"=w3989:u8, "Punkte umkehren"=w3988:bool, "zusätzliche Zeitdauer Erster Punkt"=w3987:sgl)
          }
        }
        n2127 = Unbundle By Name(w3887) -> ()  [unwired: 1 out]
        n2128 = Not Equal To 0?(x="Kalibrierauswahl") -> (x != 0?=w3927:bool)
        n2129 = property on="Start LinCheck" class="Bool."("Visible"=w3927) -> (error out=w3925:errorcluster)  [unwired: 2 in, 1 out]
        n2130 = disable-structure shown="Aktiviert" {
          disable-tunnel: "EPA Optionsfeld" -> [_ w3945]
          disable-tunnel: [EPA_Optionsfeld."Istwert" ("EPA Optionsfeld") w3945] -> w3878
          frame Enabled {
            # "#EPA_immer_Istwerte"
          }
          frame Disabled {
          }
        }
        n2131 = call <vilib>:"Clear Errors.vi"("error in (no error)"=w3925) -> ()  [unwired: 5 in, 2 out]
        n2132 = call "FGV Gasteiler.vi"("Aktionen"=Aktionen_FGV_Gasteiler_Daten."lesen") -> ("Gasteiler Daten"=w3930:T118)  [unwired: 11 in, 7 out]
        n2133 = call "aktueller SPAN und Komponent Index.vi"() -> ("akt SPAN out"=w3881:i32)  [unwired: 7 in, 4 out]
        n2134 = Unbundle By Name(w3930) -> ("Gasteiler Type"=w3905:T15)
        n2135 = Decrement(x=w3884) -> (x-1=w3880:i32)
        n2136 = call "FGV_HovaCAL_Interface_AutoLin_MFC.vi"("Aktion"=Aktion_FGV_HovaCAL_Interface_Autolin."schreiben", "AutoLin MFC"=w3908) -> ("error out"=w3892:errorcluster, "AutoLin MFC out"=w3890:u16)  [unwired: 6 in, 2 out]
        n2137 = Bundle("akt SPAN out"=w3881, w3880) -> (w3879:cluster{"akt SPAN out":i32, i32})  [unwired: 1 in]
        n2138 = call "Deaktivate HovaCAL MFC Komp fix.vi"("error in (no error)"=w3892, "AutoLin MFC"=w3890) -> ("AutoLin MFC out"=w3889:i32)  [unwired: 8 in, 1 out]
        n2139 = Equal?(x=w3905, y=w3906) -> (x = y?=w3904:bool)
        n2140 = property on="Gasnummer Generieren" class="DigWert (strikt)"("Val(Sgnl)"=w3884) -> (error out=w3893:errorcluster)  [unwired: 2 in, 1 out]
        n2141 = call "FGV Gasteiler.vi"("Aktionen"=Aktionen_FGV_Gasteiler_Daten."lesen") -> ("Anforderung"=w3933:bool)  [unwired: 11 in, 7 out]
        n2142 = call <vilib>:"Clear Errors.vi"("error in (no error)"=w3893) -> ()  [unwired: 5 in, 2 out]
        n2143 = call "EPA Polynom Ordnung je Komponente für Protokoll.vi"("Aktion"=Aktion_EPA_Polynom_Ordnung_je_Komponente_für_Protokoll."lesen", "Index in"=w3879) -> ("EPA Optionsfeld out"=w3883:T2)  [unwired: 5 in, 3 out]
        n2144 = And(x=w3933, y=w3904) -> (x .and. y?=w3907:bool)
        n2145 = Not Equal?(x=w3878, y=w3883) -> (x != y?=w3886:bool)
        n2146 = Bundle By Name(cluster=w3887, "Konfig Gasflasche"=w3919, "Gasflasche"=w3918, "Komponentenauswahl"=w3917, "Verdünnungsgas"=w3916, "Gasflaschen Nr.:"=w3915, "Bottle Accuracy"=w3914, "Bearbeiter/in"="Bearbeiter", "Messgerät"=w3910, "Gas Ablaufdatum"=w3909, "F_max gefordert (%)"=w3913, "Zeitdauer Stufe"=w3912, "Anzahl Stufen"=w3911, "EPA Optionsfeld"=w3878, "Punkte umkehren"=w3901, "Kalibrierauswahl"="Kalibrierauswahl", "Conditions:"="Conditions:", "Autolin Hovacal"=w3908, "Gasnummer:"=w3884, "Lin Modus"="Modus", "zusätzliche Zeitdauer Erster Punkt"=w3894) -> (w3942:T119)
        n2147 = case shown="True" w3886 {
          tunnel: w3878 -> [_ w3947]
          tunnel: w3879 -> [_ w3946]
          frame False {
          }
          frame True {
            # "#PDF_manu_MG"
            n2148 = call "EPA Polynom Ordnung je Komponente für Protokoll.vi"("Aktion"=Aktion_EPA_Polynom_Ordnung_je_Komponente_für_Protokoll."schreiben", "Index in"=w3946, "EPA Optionsfeld"=w3947) -> ()  [unwired: 4 in, 4 out]
          }
        }
        n2149 = control-ref of="EPA Auswertung"() -> (w3929:refnum<vi>)
        n2150 = control-ref of="Polynom-Ordnung"() -> (w3891:refnum<vi>)
        n2151 = call "Update after ProtocollParameter Changes.vi"("EPA Auswertung (Eingang)"=w3929, "Lin-Polynom"=w3942, "Polynom-Ordnung (Eingang)"=w3891) -> ("Aktiv EPA"=w3940:T57, "Stufen Tabelle"=w3897:T27, "Polynomkoeff."=w3935:T198, "EPA Ausgabetabelle"=w3939:string[][], "LIN Ausgabetabelle"=w3936:string[][], "XY-Graph"=w3938:cluster{dbl[], dbl[]}[], "LINVer Auswertung"=w3937:string[][], "Fehler (Ausgang)"=w3922:errorcluster)  [unwired: 4 in, 1 out]
        n2152 = case shown="True" w3907 {
          tunnel: w3889 -> [_ w4004]
          tunnel: w3922 -> [_ w4002]
          frame False {
          }
          frame True {
            n2153 = call "Komponentenausgabe.vi"("error in (no error)"=w4002) -> ("Konzentration"=w4005:sgl, "Gaskomponente"=w4003:T7)  [unwired: 7 in, 2 out]
            n2154 = disable-structure shown="HovaCALInterface==TRUE, Standard" {
              disable-tunnel: w4005 -> [w4007 w4028]
              disable-tunnel: w4004 -> [w4006 w4025]
              disable-tunnel: w4003 -> [_ w4026]
              frame condition #0 {
                n2155 = case shown="1" w4006 {
                  tunnel: w4007 -> [_ w4012 w4019]
                  frame 0, Default {
                  }
                  frame 1 {
